vi "call async convert tdms to png.vi"(8 "error in (no error)":errorcluster, 11 "Save Image Path":path) -> ()   [LabVIEW 2020]
uses:
  Point Grey Camera.lvclass
panel:
  # "Made reentrant"
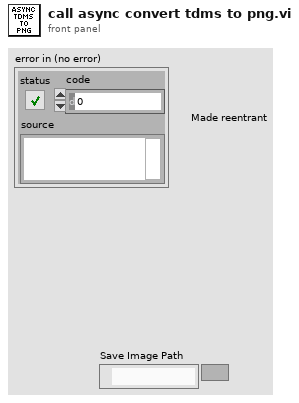
[diagram p1: front panel]
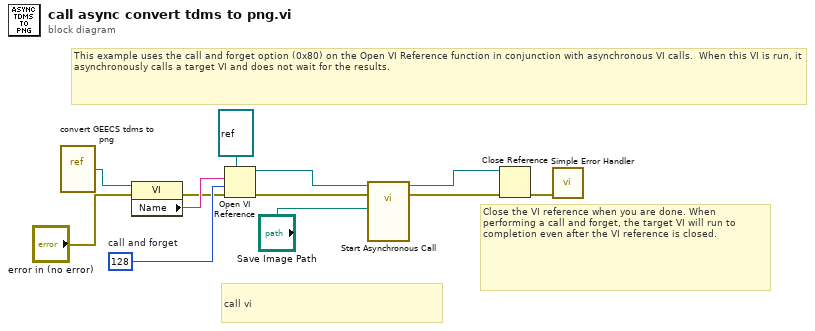
[diagram p0: block diagram]
diagram:
  w12 = 128  # call and forget
  # "This example uses the call and forget option (0x80) on the Open VI Reference function in conjunction with asynchronous VI calls.  When this VI is run, it asynchronously calls a target VI and does not wait for the results."
  # "Close the VI reference when you are done. When performing a call and forget, the target VI will run to completion even after the VI reference is closed."
  # "call vi"
  n1 = vi-ref "convert GEECS tdms to png.vi"() -> (w3:refnum<vi>)
  n2 = property class="VI"(reference=w3, error in="error in (no error)") -> (error out=w4:errorcluster, "Name"=w5:string)  [unwired: 1 out]
  n3 = Open VI Reference(type specifier VI Refnum (for type only)=refnum<vi> refnum, vi path=w5, options=w12, error in (no error)=w4) -> (vi reference=w10:refnum<vi>, error out=w9:errorcluster)  [unwired: 2 in]
  n4 = call-by-ref "Start Asynchronous Call"(reference=w10, error in=w9, "Save Image Path"="Save Image Path") -> (reference out=w7:refnum<vi>, error out=w8:errorcluster)  [unwired: 10 in, 1 out]
  n5 = Close Reference(reference=w7, error in (no error)=w8) -> (error out=w6:errorcluster)
  n6 = call "Simple Error Handler.vi"("error in (no error)"=w6) -> ()  [unwired: 4 in, 5 out]
